vi "Flush Responses.vi"(8 "error in (no error)":errorcluster, 11 "JSONRPC Server in":refnum<class "JSONRPC Server.lvclass">) -> (0 "error out":errorcluster, 3 "JSONRPC Server out":refnum<class "JSONRPC Server.lvclass">)   [LabVIEW 2015, in "JSONRPC Server.lvclass"]
uses:
  JSONRPC Server.lvclass
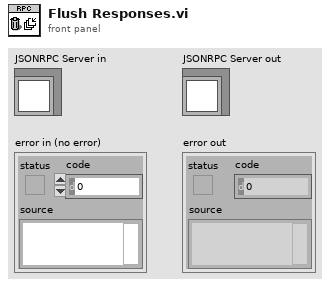
[diagram p1: front panel]
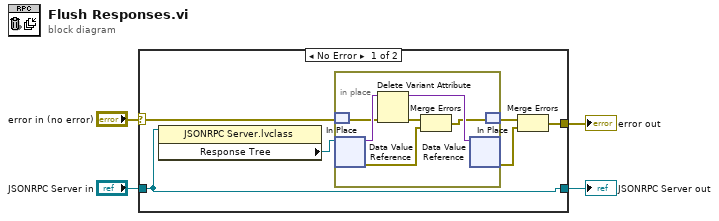
[diagram p0: block diagram]
diagram:
  n1 = case shown="No Error" "error in (no error)" {
    selector: "error in (no error)" -> [w10 w18]
    tunnel: [w9 w18] -> w3
    tunnel: [w6 w17] -> w1
    tunnel: "JSONRPC Server in" -> [w6 w17]
    frame No Error {
      n2 = property class="JSONRPC Server.lvclass"(reference=w6) -> ("Response Tree"=w5:refnum<data-value>)  [unwired: 1 in, 2 out]
      n3 = in-place {
        n4 = in-place-match #1(w10) -> (w12:errorcluster)
        n5 = in-place-dvr #2(w5) -> (w16:variant, w13:errorcluster)
        n6 = Delete Variant Attribute(4:w12, 7:w16) -> (0:w14:errorcluster, 3:w15:variant)  [unwired: 1 in, 1 out]
        n7 = Merge Errors(w14, w13) -> (w11:errorcluster)
        n8 = in-place-dvr #2(w15) -> (w7:errorcluster)  [unwired: 1 out]
        n9 = in-place-match #1(w11) -> (w8:errorcluster)
      }
      n10 = Merge Errors(w8, w7) -> (w9:errorcluster)
    }
    frame Error {
    }
  }
  "error out" <- w3
  "JSONRPC Server out" <- w1
